vi "Private Write BusMonitors.vi"(10 "BusMonitors":refnum<class "IBusMonitor.lvclass">[](array[class]), 11 "MonitoredMediator in":refnum<class "MonitoredMediator.lvclass">) -> (3 "MonitoredMediator out":refnum<class "MonitoredMediator.lvclass">)   [LabVIEW 2020, in "MonitoredMediator.lvlib" / "MonitoredMediator.lvclass"]
uses:
  <vilib>/gpm_packages/@cs/mva-core/Source/MonitoredMediator/MonitoredMediator/MonitoredMediator.lvclass
  <vilib>/gpm_packages/@cs/mva-core/Source/MonitoredMediator/IBusMonitor/IBusMonitor.lvclass
  <vilib>/gpm_packages/@cs/mva-core/Source/MonitoredMediator/MonitoredMediator/MonitoredMediator.lvclass/MonitoredMediator.ctl
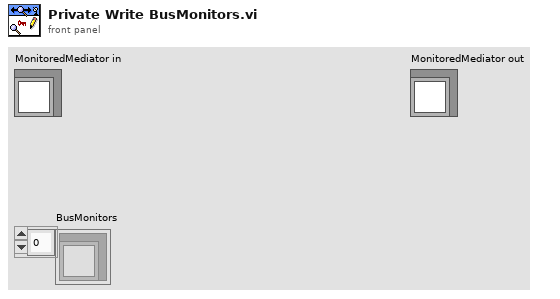
[diagram p1: front panel]
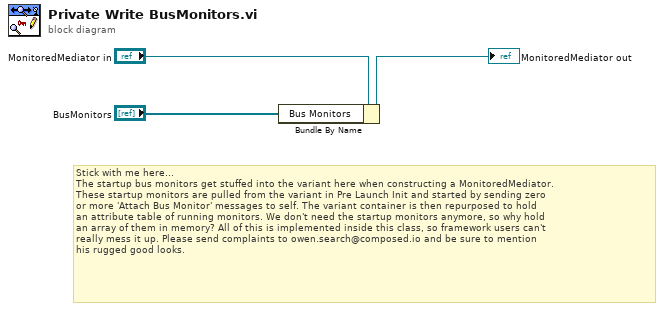
[diagram p0: block diagram]
diagram:
  # "Stick with me here...\nThe startup bus monitors get stuffed into the variant here when constructing a MonitoredMediator.\nThese startup monitors are pulled from the variant in Pre Launch Init and started by sending zero\nor more 'Attach Bus Monitor' messages to self. The variant container is then repurposed to hold\nan attribute table of running monitors. We don't need the startup monitors anymore, so why hold\nan array of them in memory? All of this is implemented inside this class, so framework users can't\nreally mess it up. Please send complaints to owen.search@composed.io and be sure to mention\nhis rugged good looks."
  n1 = Bundle By Name(cluster="MonitoredMediator in", "Bus Monitors"="BusMonitors") -> (→"MonitoredMediator out":refnum<class "MonitoredMediator.lvclass">)
